vi "Seconds to Time format.vi"(1 "No of seconds":i32) -> (0 "Time output":string)   [LabVIEW 2015, in "NI_ReportGenerationToolkit.lvlib"]
uses:
  <vilib>/addons/_office/NI_ReportGenerationToolkit.lvlib
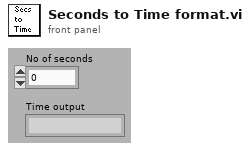
[diagram p1: front panel]
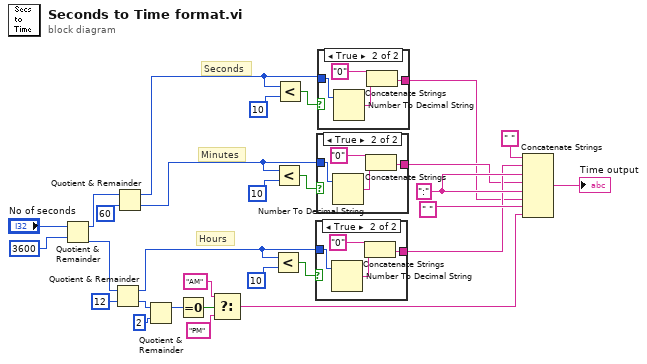
[diagram p0: block diagram]
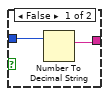
[diagram p2: hidden frame]
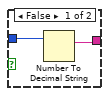
[diagram p3: hidden frame]
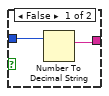
[diagram p4: hidden frame]
diagram:
  w17 = ":"
  # "Hours"
  # "Seconds"
  # "Minutes"
  n1 = Quotient & Remainder(x="No of seconds", y=3600) -> (x-y*floor(x/y)=w19:i32, floor(x/y)=w27:i32)
  n2 = Quotient & Remainder(x=w27, y=12) -> (x-y*floor(x/y)=w5:i32, floor(x/y)=w20:i32)
  n3 = Quotient & Remainder(x=w19, y=60) -> (x-y*floor(x/y)=w11:i32, floor(x/y)=w8:i32)
  n4 = Quotient & Remainder(x=w20, y=2) -> (x-y*floor(x/y)=w24:i32)  [unwired: 1 out]
  n5 = Equal To 0?(x=w24) -> (x = 0?=w23:bool)
  n6 = Select(t="AM", s=w23, f="PM") -> (s? t:f=w4:string)
  n7 = Less?(x=w5, y=10) -> (x < y?=w6:bool)
  n8 = Less?(x=w8, y=10) -> (x < y?=w9:bool)
  n9 = Less?(x=w11, y=10) -> (x < y?=w12:bool)
  n10 = case shown="True" w6 {
    tunnel: w5 -> [w31 w34]
    tunnel: [w30 w32] -> w3
    frame False {
      n11 = Number To Decimal String(number=w31) -> (decimal integer string=w30:string)  [unwired: 1 in]
    }
    frame True {
      n12 = Number To Decimal String(number=w34) -> (decimal integer string=w33:string)  [unwired: 1 in]
      n13 = Concatenate Strings("0", w33) -> (w32:string)
    }
  }
  n14 = case shown="True" w9 {
    tunnel: w8 -> [w37 w40]
    tunnel: [w36 w38] -> w2
    frame False {
      n15 = Number To Decimal String(number=w37) -> (decimal integer string=w36:string)  [unwired: 1 in]
    }
    frame True {
      n16 = Number To Decimal String(number=w40) -> (decimal integer string=w39:string)  [unwired: 1 in]
      n17 = Concatenate Strings("0", w39) -> (w38:string)
    }
  }
  n18 = case shown="True" w12 {
    tunnel: w11 -> [w43 w46]
    tunnel: [w42 w44] -> w1
    frame False {
      n19 = Number To Decimal String(number=w43) -> (decimal integer string=w42:string)  [unwired: 1 in]
    }
    frame True {
      n20 = Number To Decimal String(number=w46) -> (decimal integer string=w45:string)  [unwired: 1 in]
      n21 = Concatenate Strings("0", w45) -> (w44:string)
    }
  }
  n22 = Concatenate Strings(" ", w3, w17, w2, w17, w1, " ", w4) -> (→"Time output":string)
